vi "Off laser.vi"() -> ()   [LabVIEW 2010]
panel:
  in  "wait(min)":i32
  in  "Laser GPIB":u8=10 max=100
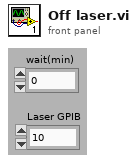
[diagram p1: front panel]
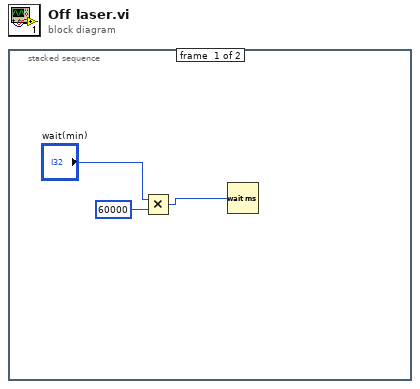
[diagram p0: block diagram]
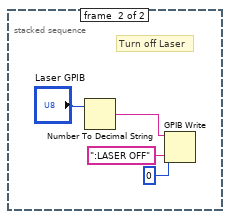
[diagram p2: hidden frame]
diagram:
  n1 = stacked-sequence {
    frame #0 {
      n2 = Multiply(x="wait(min)", y=60000) -> (x*y=w1:i32)
      n3 = Wait (ms)(milliseconds to wait=w1) -> ()  [unwired: 1 out]
    }
    frame #1 {
      # "Turn off Laser"
      n4 = Number To Decimal String(number="Laser GPIB") -> (decimal integer string=w4:string)  [unwired: 1 in]
      n5 = GPIB Write(0:w4, 1:":LASER OFF" ("data"), 2:i16 0 ("mode (0)")) -> ()  [unwired: 2 in, 2 out]
    }
  }
